vi "Motion@SetTool__Parameter.vi"(1 "ParamterIn":string) -> (0 "ParamterOut":string)   [LabVIEW 2020]
panel:
  in  "PreTool":string(combo)
  in  "PointName":string(combo)
  in  "MotorName":string(combo)
  in  "Confirm":bool
  # "Motion@SetTool $Motor,$Point(@XYZUVW,$PreTool)\nMotion@SetTool $Motor,(x,y,z,u)(,$PreTool)\nMotion@SetTool $Motor,(x,y,inf,inf)(,$PreTool)  --> set XY only, keep z,u\nMotion@SetTool $Motor   --> Reset to Default Value (0,0,0,0)"
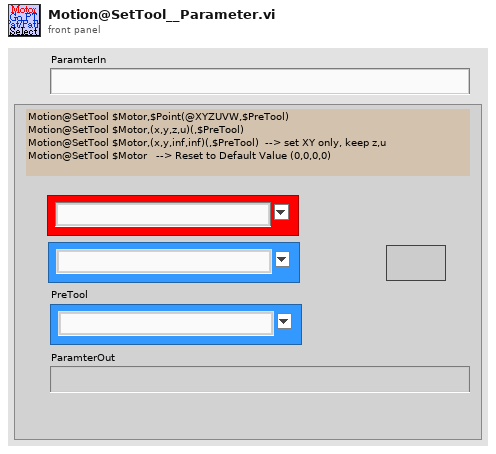
[diagram p1: front panel]
types:
  T1 = enum16{"Get", "UpdatePointS", "Init", "UpdateIndex", "GetCurrent&Index+1", "GetWithIndex", "ChkLast", "GetCurrent"}
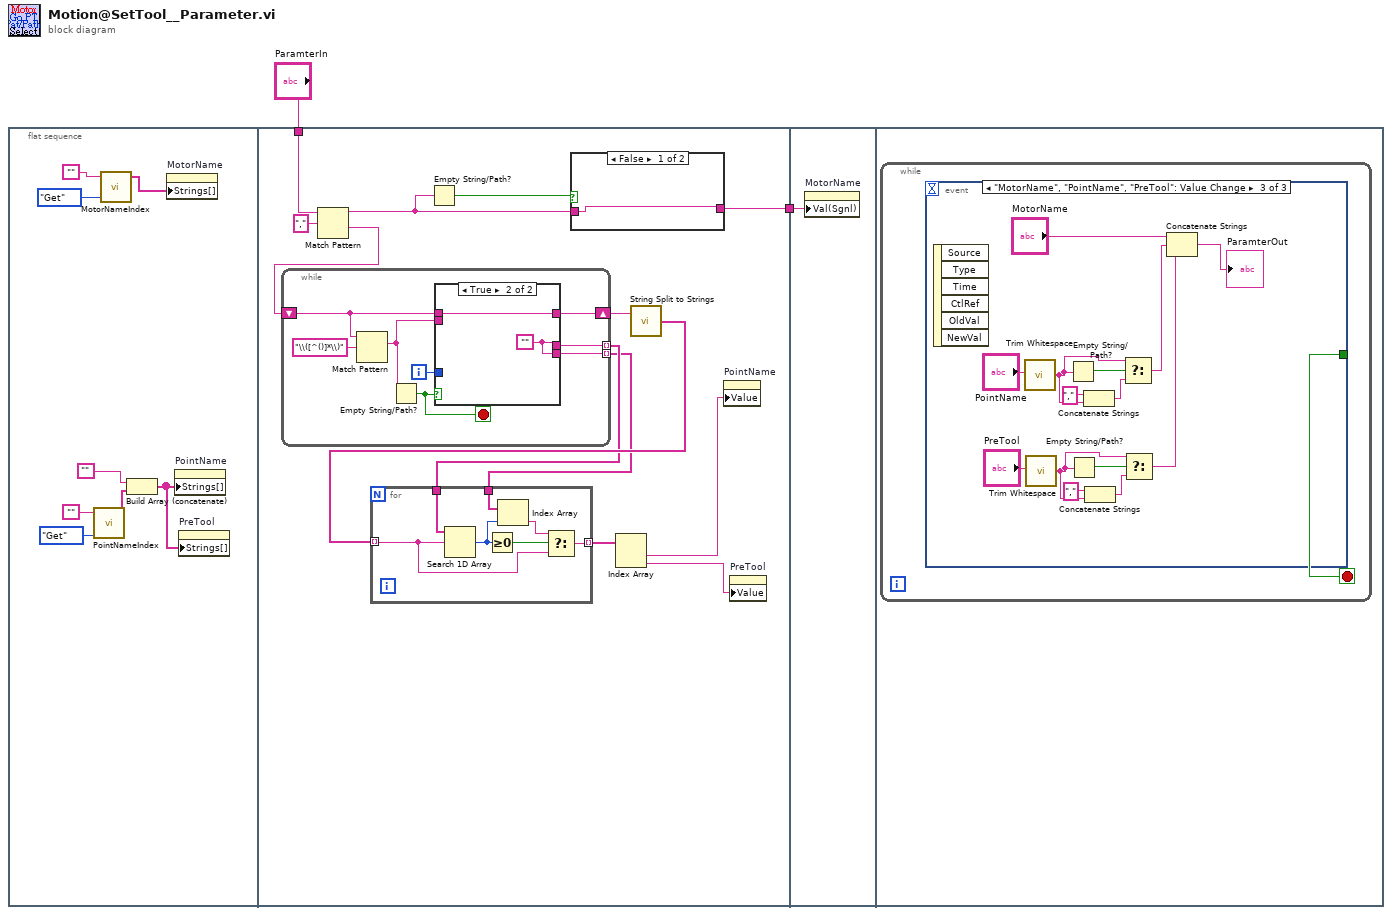
[diagram p0: block diagram]
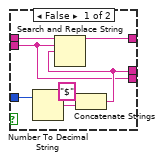
[diagram p2: hidden frame]
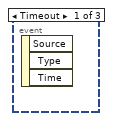
[diagram p4: hidden frame]
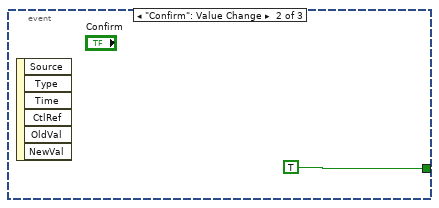
[diagram p5: hidden frame]
diagram:
  n1 = flat-sequence {
    tunnel: "ParamterIn" -> [w22]
    tunnel: [w19] -> w1
    tunnel: w1 -> [w50]
    frame #0 {
      n2 = call "PointNameIndex.vi"("OP"=T1."Get", "PointName"="") -> ("PointNameList"=w4:string[])  [unwired: 4 in, 5 out]
      n3 = call "MotorNameIndex.vi"("OP"=enum16{"Get", "Update", "Init"}."Get", "MotorName"="") -> ("MotorList"=w8:string[])  [unwired: 1 in, 2 out]
      n4 = Build Array (concatenate)("", w4) -> (w3:string[])
      n5 = property on="MotorName" class="CmbBox"("Strings[]"=w8) -> ()  [unwired: 2 in, 2 out]
      n6 = property on="PointName" class="CmbBox"("Strings[]"=w3) -> ()  [unwired: 2 in, 2 out]
      n7 = property on="PreTool" class="CmbBox"("Strings[]"=w3) -> ()  [unwired: 2 in, 2 out]
    }
    frame #1 {
      n8 = Match Pattern(string=w22, regular expression=",") -> (before substring=w20:string, after substring=w18:string)  [unwired: 1 in, 2 out]
      n9 = while {
        shift-right: [w35] -> w17
        shift-left: w18 -> [w33]
        tunnel: [w32] -> w15 mode=indexing
        tunnel: [w31] -> w14 mode=indexing
        i -> [w34]
        stop <- w36 stop-if-true
        n10 = Match Pattern(string=w33, regular expression="\\([^()]*\\)") -> (match substring=w37:string)  [unwired: 1 in, 3 out]
        n11 = Empty String/Path?(string/path=w37) -> (empty?=w36:bool)
        n12 = case shown="True" w36 {
          tunnel: w33 -> [w45 w47]
          tunnel: w37 -> [w39 _]
          tunnel: [w44 w47] -> w35
          tunnel: w34 -> [w41 _]
          tunnel: [w40 w46] -> w32
          tunnel: [w39 w46] -> w31
          frame False {
            n13 = Number To Decimal String(number=w41) -> (decimal integer string=w43:string)  [unwired: 1 in]
            n14 = Concatenate Strings("$" ("string"), w43) -> (w40:string)
            n15 = Search and Replace String(input string=w45, search string=w39, replace string=w40) -> (result string=w44:string)  [unwired: 5 in, 3 out]
          }
          frame True {
            w46 = ""
          }
        }
      }
      n16 = Empty String/Path?(string/path=w20) -> (empty?=w23:bool)
      n17 = case shown="False" w23 {
        tunnel: w20 -> [w48 w49]
        tunnel: [w48 w49] -> w19
        frame False {
        }
        frame True {
        }
      }
      n18 = call "String Split to Strings.vi"("String"=w17) -> ("Array"=w16:string[])  [unwired: 1 in]
      n19 = for {
        tunnel: w16 -> [w28] mode=indexing
        tunnel: w15 -> [w30]
        tunnel: w14 -> [w27]
        tunnel: [w24] -> w13 mode=indexing
        n20 = Search 1D Array(1D array=w30, element=w28) -> (index of element=w26:i32)  [unwired: 1 in]
        n21 = Greater Or Equal To 0?(x=w26) -> (x >= 0?=w29:bool)
        n22 = Index Array(array=w27, index=w26) -> (element=w25:string)
        n23 = Select(t=w25, s=w29, f=w28) -> (s? t:f=w24:string)
      }
      n24 = Index Array(array=w13) -> (element #1=w12:string, element #2=w11:string)  [unwired: 2 in]
      n25 = property on="PointName" class="CmbBox"("Value"=w12) -> ()  [unwired: 2 in, 2 out]
      n26 = property on="PreTool" class="CmbBox"("Value"=w11) -> ()  [unwired: 2 in, 2 out]
    }
    frame #2 {
      n27 = property on="MotorName" class="CmbBox"("Val(Sgnl)"=w50) -> ()  [unwired: 2 in, 2 out]
    }
    frame #3 {
      n28 = while {
        stop <- w51 stop-if-true
        n29 = event shown="[2] \"MotorName\", \"PointName\", \"PreTool\": Value Change" {
          selector: _ -> [_ _ _]
          dyn-events: _ -> [_ _ _]
          timeout: _ -> [_ _ _]
          tunnel: [_ TRUE _] -> w51
          event Timeout {
            n30 = event-data() -> ()  [unwired: 1 in, 3 out]
          }
          event "Confirm": Value Change {
            n31 = event-data() -> ()  [unwired: 1 in, 6 out]
          }
          event "MotorName", "PointName", "PreTool": Value Change {
            n32 = event-data() -> ()  [unwired: 1 in, 6 out]
            n33 = call <vilib>:"Trim Whitespace.vi"("string"="PointName") -> ("trimmed string"=w61:string)  [unwired: 1 in]
            n34 = call <vilib>:"Trim Whitespace.vi"("string"="PreTool") -> ("trimmed string"=w57:string)  [unwired: 1 in]
            n35 = Empty String/Path?(string/path=w61) -> (empty?=w64:bool)
            n36 = Empty String/Path?(string/path=w57) -> (empty?=w54:bool)
            n37 = Concatenate Strings("," ("string"), w61) -> (w60:string)
            n38 = Concatenate Strings("," ("string"), w57) -> (w58:string)
            n39 = Select(t=w61, s=w64, f=w60) -> (s? t:f=w59:string)
            n40 = Select(t=w57, s=w54, f=w58) -> (s? t:f=w53:string)
            n41 = Concatenate Strings("MotorName", w59, w53) -> (→"ParamterOut":string)
          }
        }
      }
    }
  }
